vi "tearDown.vi"(8 "error in (no error)":errorcluster, 11 "reference in":refnum<class "Telemetry System Tests.lvclass">) -> (0 "error out":errorcluster, 3 "reference out":refnum<class "Telemetry System Tests.lvclass">)   [LabVIEW 2019, in "Telemetry System Tests.lvclass"]
doc: "tearDown runs after the test method has completed. Use this method to clean up any operations or references that were opened by setUp or the test method. Unit tests should be independent of other unit tests so this VI should ensure that the next test can run in a 'clean' test environment."
uses:
  Telemetry System Tests.lvclass
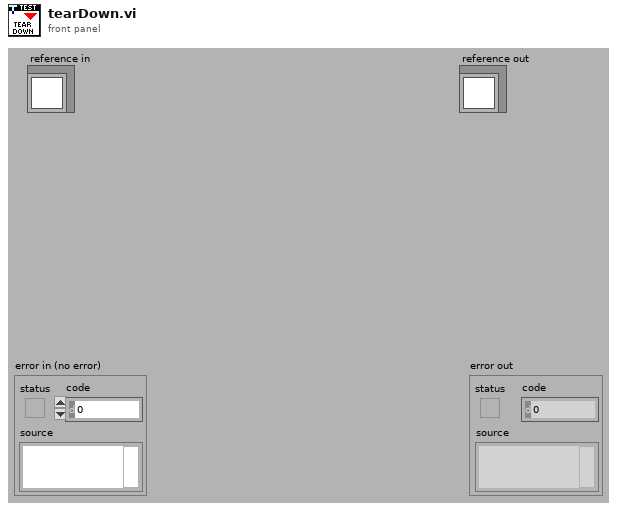
[diagram p1: front panel]
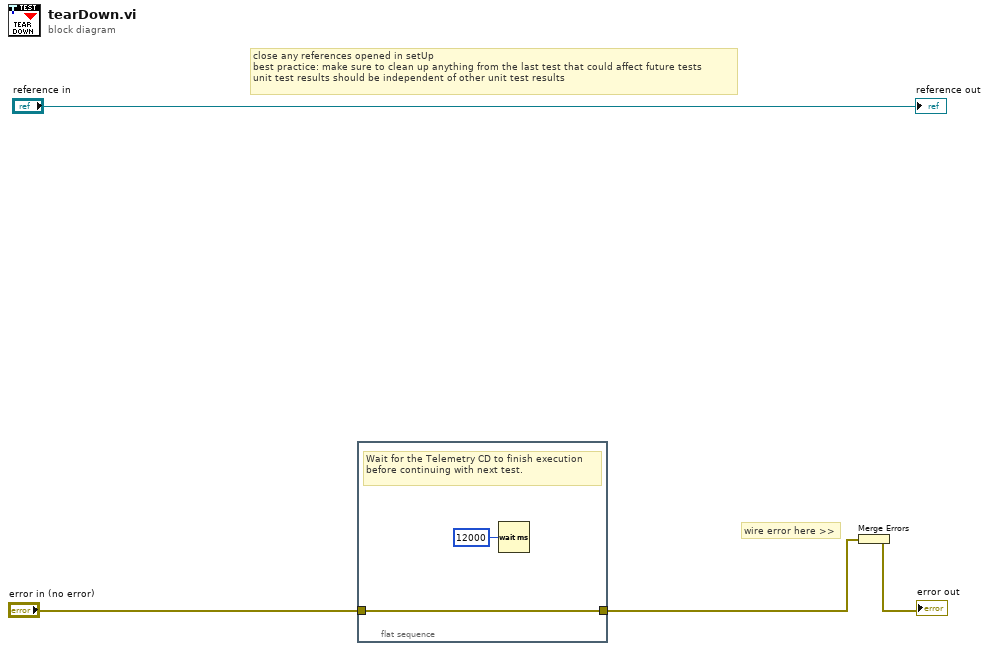
[diagram p0: block diagram]
diagram:
  # "wire error here >>"
  # "close any references opened in setUp\nbest practice: make sure to clean up anything from the last test that could affect future tests\nunit test results should be independent of other unit test results"
  n1 = flat-sequence {
    tunnel: "error in (no error)" -> [w5]
    tunnel: [w5] -> w1
    frame #0 {
      # "Wait for the Telemetry CD to finish execution before continuing with next test."
      n2 = Wait (ms)(milliseconds to wait=u32 12000) -> ()  [unwired: 1 out]
    }
  }
  n3 = Merge Errors(w1) -> (→"error out":errorcluster)
  "reference out" <- "reference in"
